vi "read_all_config_keys.vi"(8 "error_in":errorcluster, 11 "config_file_path":path) -> (0 "error_out":errorcluster, 3 "config_info":T1)   [LabVIEW 2020]
uses:
  config_info.ctl
  <vilib>/Utility/config.llb/Read Key (String).vi
  <vilib>/Utility/config.llb/NI_LVConfig.lvlib
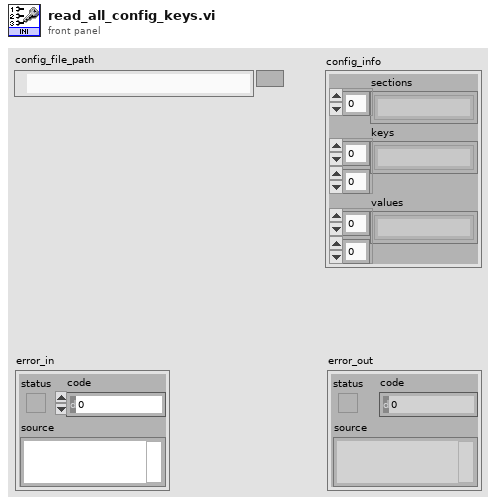
[diagram p1: front panel]
types:
  T1 = typedef "config_info.ctl" = cluster{"sections":string[], "keys":string[][], "values":string[][]}
  T2 = typedef "NI_LVConfig.lvlib/Config Data RefNum.ctl" = refnum<k1>
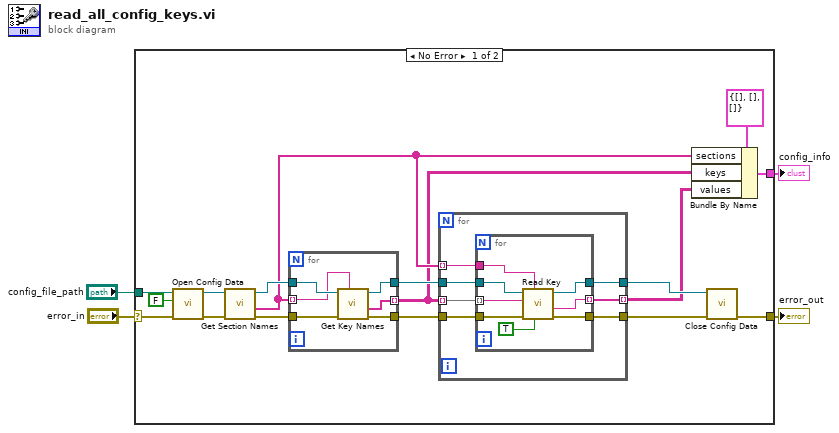
[diagram p0: block diagram]
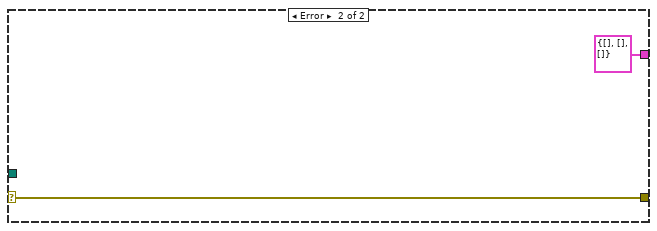
[diagram p2: hidden frame]
diagram:
  n1 = case shown="No Error" "error_in" {
    selector: "error_in" -> [w6 w44]
    tunnel: "config_file_path" -> [w17 _]
    tunnel: [w12 w44] -> w3
    tunnel: [w7 T1 {"sections"=[], "keys"=[], "values"=[]} ("input cluster")] -> w2
    frame No Error {
      n2 = call <vilib>:"Open Config Data.vi"("error in (no error)"=w6, "create file if necessary (T)"=FALSE, "configuration file path"=w17) -> ("error out"=w21:errorcluster, "refnum"=w20:T2)  [unwired: 6 in, 1 out]
      n3 = call <vilib>:"Get Section Names.vi"("error in (no error)"=w21, "refnum"=w20) -> ("error out"=w18:errorcluster, "section names"=w10:string[], "refnum out"=w19:T2)  [unwired: 7 in]
      n4 = for {
        tunnel: w19 -> [w42]
        tunnel: w18 -> [w41]
        tunnel: [w38] -> w15
        tunnel: [w40] -> w16
        tunnel: w10 -> [w39] mode=indexing
        tunnel: [w37] -> w9 mode=indexing
        n5 = call <vilib>:"Get Key Names.vi"("section"=w39, "error in (no error)"=w41, "refnum"=w42) -> ("error out"=w38:errorcluster, "key names"=w37:string[], "refnum out"=w40:T2)  [unwired: 5 in, 1 out]
      }
      n6 = for {
        tunnel: w16 -> [w27]
        tunnel: w15 -> [w28]
        tunnel: w10 -> [w26] mode=indexing
        tunnel: w9 -> [w25] mode=indexing
        tunnel: [w23] -> w14
        tunnel: [w22] -> w13
        tunnel: [w24] -> w8 mode=indexing
        n7 = for {
          tunnel: w27 -> [w35]
          tunnel: w26 -> [w36]
          tunnel: w25 -> [w34] mode=indexing
          tunnel: w28 -> [w33]
          tunnel: [w32] -> w23
          tunnel: [w31] -> w22
          tunnel: [w30] -> w24 mode=indexing
          n8 = call-poly <vilib>:"Read Key.vi"("read raw string? (F)"=TRUE, "section"=w36, "error in (no error)"=w33, "key"=w34, "refnum"=w35) -> ("error out"=w31:errorcluster, "value"=w30:string, "refnum out"=w32:T2)  [unwired: 3 in, 1 out]
        }
      }
      n9 = Bundle By Name(cluster=T1 {"sections"=[], "keys"=[], "values"=[]} ("input cluster"), "sections"=w10, "keys"=w9, "values"=w8) -> (w7:T1)
      n10 = call <vilib>:"Close Config Data.vi"("error in (no error)"=w13, "refnum"=w14) -> ("error out"=w12:errorcluster)  [unwired: 8 in, 1 out]
    }
    frame Error {
    }
  }
  "error_out" <- w3
  "config_info" <- w2
